vi "ExSubCollectDisplayStore.vi"(3 "error in (no error)":errorcluster, 4 "Store flag":i8, 5 "Display Title":string, 6 "Handle Cluster":T1) -> (0 "error out":errorcluster, 1 "got frame":u32, 2 "Handle Cluster Out":T1)   [LabVIEW 2010]
panel:
  # "ExSubCollectDisplayStore:\nThis sub-VI checks to see if data has arrived from camera,\nif so it then puts it in image object and displays it. If store \nswitch is set it will also store it."
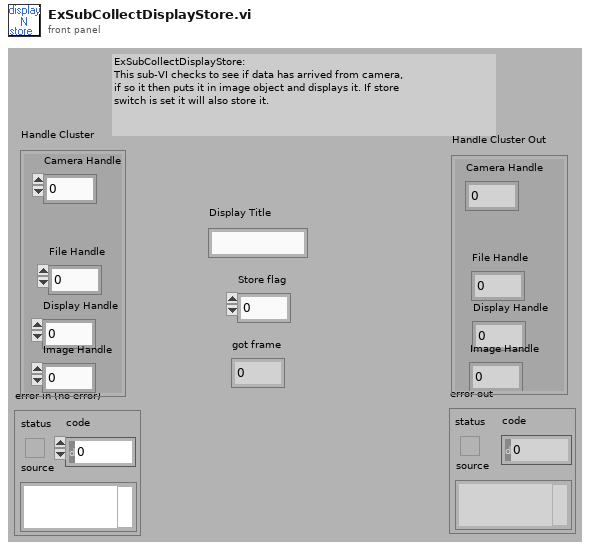
[diagram p1: front panel]
types:
  T1 = cluster{"Camera Handle":u32, "File Handle":u32, "Display Handle":u32, "Image Handle":u32}
  T2 = cluster{"Camera Handle":u32, "File Handle":u32, "Display Handle":u32, "Data Handle":u32}
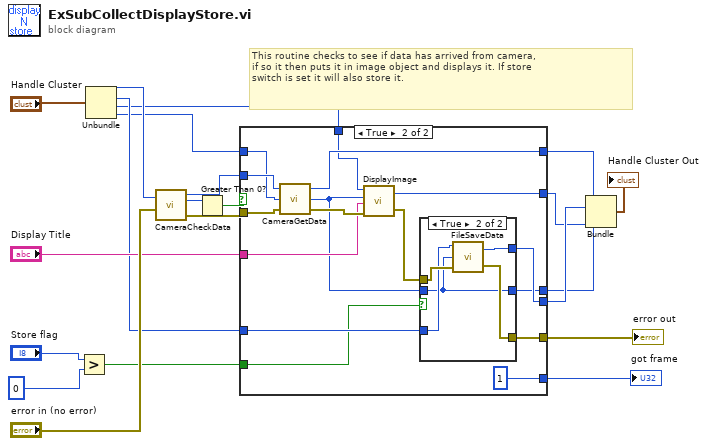
[diagram p0: block diagram]
diagram:
  # "This routine checks to see if data has arrived from camera,\nif so it then puts it in image object and displays it. If store \nswitch is set it will also store it."
  n1 = Greater?(x="Store flag", y=0) -> (0:w5:bool)
  n2 = Unbundle("Handle Cluster") -> ("Camera Handle"=w11:u32, "File Handle"=w3:u32, "Display Handle"=w2:u32, "Image Handle"=w1:u32)
  n3 = call <userlib>:"CameraCheckData.vi"("Camera Handle"=w11, "error in"="error in (no error)") -> ("Camera Handle"=w18:u32, "Number Of Frames Available"=w17:i32, "error out"=w16:errorcluster)
  n4 = Greater Than 0?(x=w17) -> (x > 0?=w19:bool)
  n5 = case shown="True" w19 {
    tunnel: w18 -> [w27 w43]
    tunnel: w16 -> [w26 w42]
    tunnel: w1 -> [w23 w37]
    tunnel: w2 -> [w25 w36]
    tunnel: [w27 w41] -> w12
    tunnel: [w24 w40] -> w10
    tunnel: "Display Title" -> [_ w35]
    tunnel: w3 -> [w24 w34]
    tunnel: [w25 w33] -> w9
    tunnel: [w26 w32] -> w13
    tunnel: [w23 w30] -> w8
    tunnel: w5 -> [_ w29]
    tunnel: [0 1] -> w4
    frame False {
    }
    frame True {
      n6 = call <userlib>:"CameraGetData.vi"("error in"=w42, "Data Handle"=w37, "Camera Handle"=w43) -> ("error out"=w39:errorcluster, "Data Handle"=w31:u32, "Camera Handle"=w41:u32)
      n7 = call <userlib>:"DisplayImage.vi"("error in"=w39, "Title"=w35, "Image Handle"=w31, "Display Handle"=w36) -> ("error out"=w38:errorcluster, "Display Handle"=w33:u32)
      n8 = case shown="True" w29 {
        tunnel: [w46 w51] -> w40
        tunnel: w38 -> [w45 w50]
        tunnel: w34 -> [w46 w48]
        tunnel: [w45 w49] -> w32
        tunnel: w31 -> [w44 w47]
        tunnel: [w44 w47] -> w30
        frame False {
        }
        frame True {
          n9 = call <userlib>:"FileSaveData.vi"("error in"=w50, "Image Handle"=w47, "File Handle"=w48) -> ("error out"=w49:errorcluster, "File Handle"=w51:u32)
        }
      }
    }
  }
  "error out" <- w13
  "got frame" <- w4
  n10 = Bundle("Camera Handle"=w12, "File Handle"=w10, "Display Handle"=w9, "Data Handle"=w8) -> (→"Handle Cluster Out":T2)  [unwired: 1 in]
